vi "set_control_refs.vi"(8 "error in (no error)":errorcluster, 10 "control refs":T1, 11 "StimulatorAK101022TCP in":refnum<class "StimulatorAK101022TCP.lvclass">) -> (0 "error out":errorcluster, 3 "StimulatorAK101022TCP out":refnum<class "StimulatorAK101022TCP.lvclass">)   [LabVIEW 2010, in "StimulatorAK101022TCP.lvclass"]
uses:
  StimulatorAK101022TCP.lvclass
  control_refs_cluster.ctl
  class_data.vi
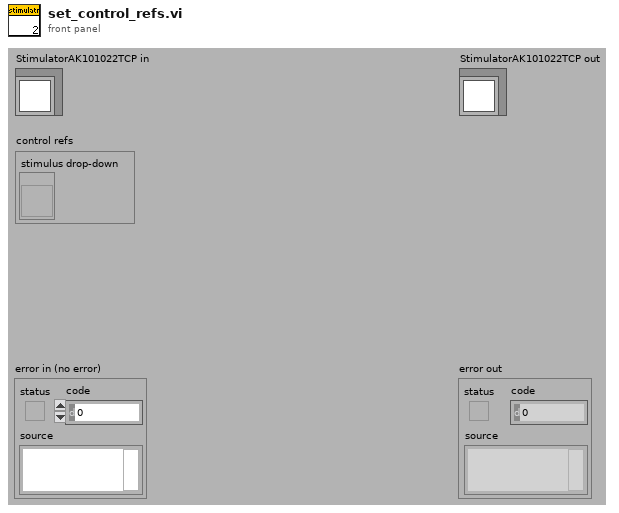
[diagram p1: front panel]
types:
  T1 = typedef "StimulatorAK101022TCP.lvclass/control_refs_cluster.ctl" = cluster{"stimulus drop-down":refnum<vi>}
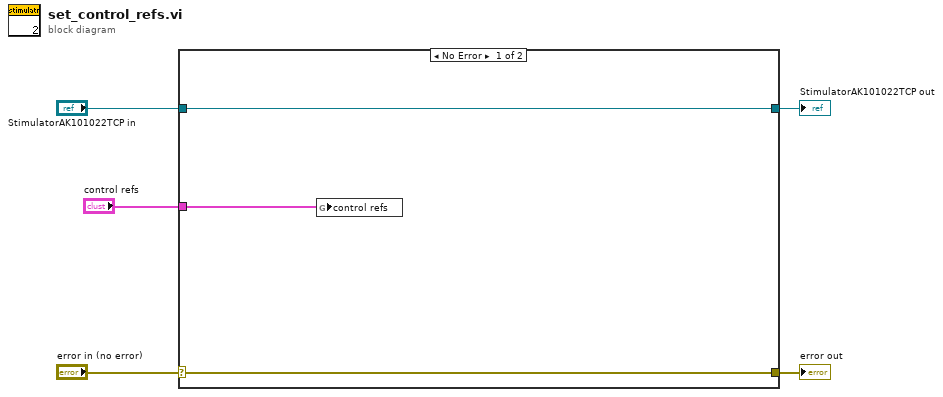
[diagram p0: block diagram]
diagram:
  n1 = case shown="No Error" "error in (no error)" {
    selector: "error in (no error)" -> [w7 w10]
    tunnel: [w7 w10] -> w4
    tunnel: [w8 w9] -> w2
    tunnel: "StimulatorAK101022TCP in" -> [w8 w9]
    tunnel: "control refs" -> [w6 _]
    frame No Error {
      n2 = global write "class_data.vi" "control refs"(w6) -> ()
    }
    frame Error {
    }
  }
  "error out" <- w4
  "StimulatorAK101022TCP out" <- w2
